vi "Temperature read and control.vi"() -> ()   [LabVIEW 2019]
uses:
  <vilib>/Utility/file.llb/Write Delimited Spreadsheet (DBL).vi
panel:
  in  "Range 2":string(combo)="HI"
  in  "Range1":string(combo)="HI"
  in  "?":enum32{"选项卡 1", "选项卡 2"}(tab)
  out "XY图":cluster{"X":dbl[], "Y":dbl[]}[](graph)
  out "XY图 2":cluster{"X":dbl[], "Y":dbl[]}[](graph)
  in  "EXIT":bool
  in  "LOOP2":dbl=273.15
  out "CHD":dbl
  out "CHC":dbl
  out "CHB":dbl
  in  "控温":bool
  in  "LOOP1":dbl=273.15
  in  "仪器地址":refnum<visa-resource-name>="tcpip0::192.168.1.5::5000::SOCKET"
  out "CHA":dbl
  in  "Delay Time (s)":i32=2 caption="延迟时间(s)"
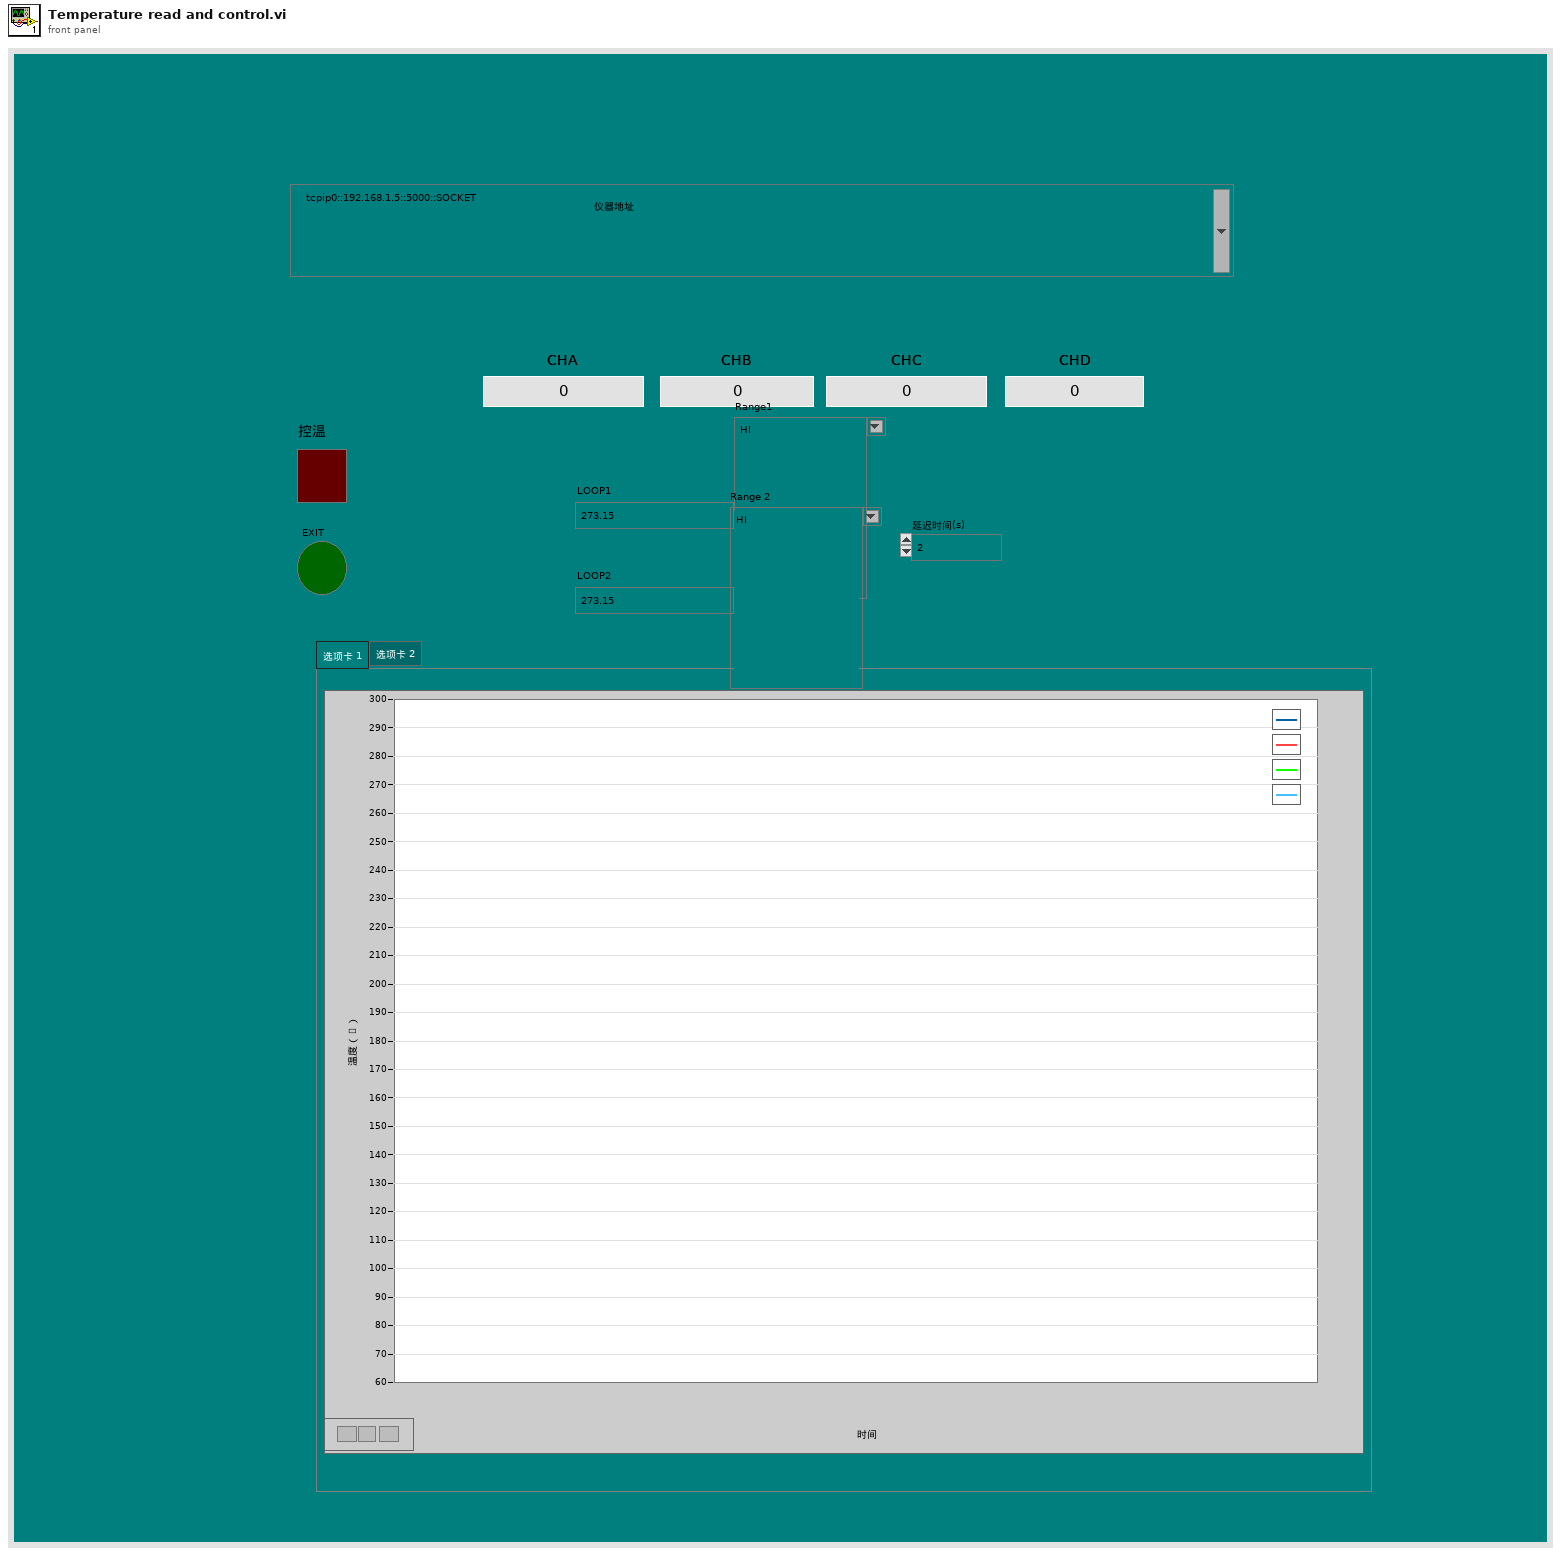
[diagram p1: front panel]
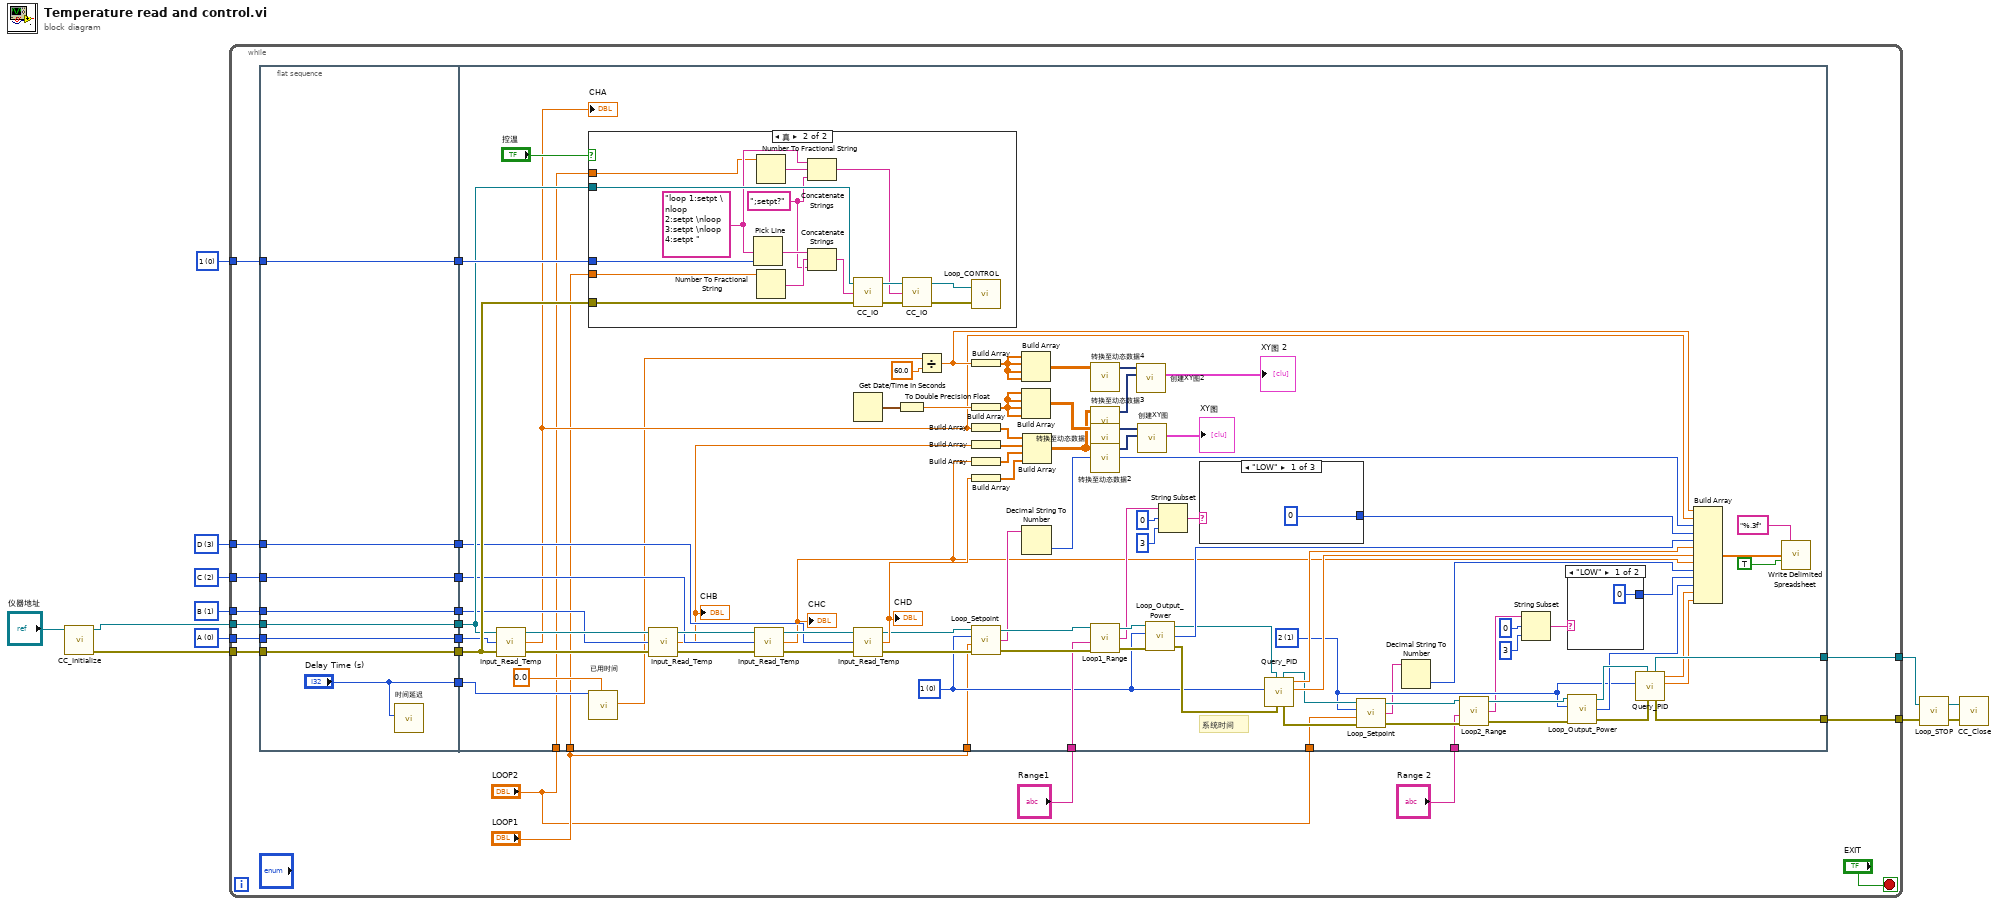
[diagram p0: block diagram]
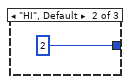
[diagram p2: hidden frame]
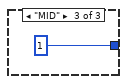
[diagram p3: hidden frame]
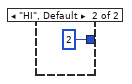
[diagram p4: hidden frame]
diagram:
  w4 = u8 3 items=["A", "B", "C", "D"] ("Input")
  w5 = u8 2 items=["A", "B", "C", "D"] ("Input")
  w6 = u8 1 items=["A", "B", "C", "D"] ("Input")
  w7 = u8 0 items=["A", "B", "C", "D"] ("Input")
  w8 = u8 0 items=["1", "2", "3", "4"] ("Loop")
  n1 = call "CC_Initialize.vi"("VISA resource name"="仪器地址") -> ("error out"=w2:errorcluster, "VISA resource name out"=w3:refnum<visa-resource-name>)  [unwired: 9 in]
  n2 = while {
    tunnel: [w29] -> w11
    tunnel: [w28] -> w12
    tunnel: w3 -> [w30]
    tunnel: w2 -> [w33]
    tunnel: w8 -> [w32]
    tunnel: w7 -> [w31]
    tunnel: w6 -> [w27]
    tunnel: w5 -> [w26]
    tunnel: w4 -> [w25]
    stop <- "EXIT" stop-if-true
    n3 = flat-sequence {
      tunnel: w25 -> [w36]
      tunnel: w26 -> [w37]
      tunnel: w27 -> [w38]
      tunnel: w30 -> [w39]
      tunnel: w31 -> [w40]
      tunnel: w32 -> [w41]
      tunnel: w33 -> [w42]
      tunnel: [w42] -> w24
      tunnel: [w41] -> w23
      tunnel: [w40] -> w22
      tunnel: [w39] -> w21
      tunnel: [w38] -> w20
      tunnel: [w37] -> w19
      tunnel: [w36] -> w18
      tunnel: ["Delay Time (s)"] -> w17
      tunnel: [w76] -> w29
      tunnel: [w75] -> w28
      tunnel: w24 -> [w129]
      tunnel: w23 -> [w128]
      tunnel: w22 -> [w127]
      tunnel: w21 -> [w126]
      tunnel: w20 -> [w119]
      tunnel: w19 -> [w118]
      tunnel: w18 -> [w117]
      tunnel: w17 -> [w99]
      tunnel: "Range1" -> [w86]
      tunnel: "Range 2" -> [w70]
      tunnel: "LOOP2" -> [w48]
      tunnel: "LOOP1" -> [w47]
      tunnel: "LOOP1" -> [w46]
      tunnel: "LOOP2" -> [w45]
      frame #0 {
        n4 = call "时间延迟"("Delay Time (s)"="Delay Time (s)") -> ()  [unwired: 10 in, 1 out]
      }
      frame #1 {
        w65 = u8 1 items=["1", "2", "3", "4"] ("Loop")
        w66 = u8 0 items=["1", "2", "3", "4"] ("Loop")
        # "系统时间"
        n5 = call "Input_Read_Temp.vi"("error in (no error)"=w129, "Input"=w127, "VISA In"=w126) -> ("error out"=w124:errorcluster, "Temperature"=w93:dbl, "VISA Out"=w125:refnum<visa-resource-name>)
        "CHA" <- w93
        n6 = case shown="真" "控温" {
          tunnel: w126 -> [_ w147]
          tunnel: w129 -> [_ w148]
          tunnel: w128 -> [_ w149]
          tunnel: w48 -> [_ w138]
          tunnel: w47 -> [_ w137]
          frame False {
          }
          frame True {
            w145 = ";setpt?" ("string")
            w144 = "loop 1:setpt \nloop 2:setpt \nloop 3:setpt \nloop 4:setpt " ("string")
            n7 = Pick Line(multi-line string=w144, line index=w149) -> (output string=w150:string)  [unwired: 1 in]
            n8 = Number To Fractional String(number=w138) -> (F-format string=w146:string)  [unwired: 3 out]
            n9 = Number To Fractional String(number=w137) -> (F-format string=w151:string)  [unwired: 3 out]
            n10 = Concatenate Strings(w144, w146, w145) -> (w139:string)
            n11 = Concatenate Strings(w150, w151, w145) -> (w152:string)
            n12 = call "CC_IO.vi"("error in (no error)"=w148, "Output Command"=w152, "VISA In"=w147) -> ("error out"=w143:errorcluster, "VISA out"=w142:refnum<visa-resource-name>)  [unwired: 1 out]
            n13 = call "CC_IO.vi"("error in (no error)"=w143, "Output Command"=w139, "VISA In"=w142) -> ("error out"=w140:errorcluster, "VISA out"=w141:refnum<visa-resource-name>)  [unwired: 1 out]
            n14 = call "Loop_CONTROL.vi"("error in (no error)"=w140, "VISA In"=w141) -> ()  [unwired: 2 out]
          }
        }
        n15 = call "已用时间"("Time Target (s)"=w99, "Set Start Time (s)"=0.0) -> ("Elapsed Time (s)"=w63:dbl)  [unwired: 10 in, 7 out]
        n16 = call "Input_Read_Temp.vi"("error in (no error)"=w124, "Input"=w119, "VISA In"=w125) -> ("error out"=w122:errorcluster, "Temperature"=w43:dbl, "VISA Out"=w123:refnum<visa-resource-name>)
        "CHB" <- w43
        n17 = call "Input_Read_Temp.vi"("error in (no error)"=w122, "Input"=w118, "VISA In"=w123) -> ("error out"=w120:errorcluster, "Temperature"=w44:dbl, "VISA Out"=w121:refnum<visa-resource-name>)
        "CHC" <- w44
        n18 = Get Date/Time In Seconds() -> (seconds since 1Jan1904=w131:timestamp)
        n19 = call "Input_Read_Temp.vi"("error in (no error)"=w120, "Input"=w117, "VISA In"=w121) -> ("error out"=w92:errorcluster, "Temperature"=w114:dbl, "VISA Out"=w91:refnum<visa-resource-name>)
        "CHD" <- w114
        n20 = To Double Precision Float(number=w131) -> (double precision float=w109:dbl)
        n21 = Divide(x=w63, y=60.0) -> (x/y=w94:dbl)
        n22 = Build Array(w94) -> (w102:dbl[])
        n23 = Build Array(w109) -> (w108:dbl[])
        n24 = Build Array(w93) -> (w113:dbl[])
        n25 = Build Array(w43) -> (w112:dbl[])
        n26 = Build Array(w44) -> (w111:dbl[])
        n27 = Build Array(w114) -> (w110:dbl[])
        n28 = call "Loop_Setpoint.vi"("VISA in"=w91, "Loop"=w66, "Setpoint"=w46, "error in"=w92) -> ("VISA out"=w90:refnum<visa-resource-name>, "Return"=w62:string, "ErrorOut"=w89:errorcluster)  [unwired: 1 in]
        n29 = Build Array(w102, w102, w102, w102) -> (w103:dbl[][])
        n30 = Build Array(w108, w108, w108, w108) -> (w107:dbl[][])
        n31 = Decimal String To Number(string=w62) -> (number=w61:i32)  [unwired: 2 in, 1 out]
        n32 = Build Array(w113, w112, w111, w110) -> (w104:dbl[][])
        n33 = call "转换至动态数据4"("2D Array"=w103) -> ("Dynamic Data Type"=w105:dynamicdata)  [unwired: 3 in]
        n34 = call "转换至动态数据3"("2D Array"=w104) -> ("Dynamic Data Type"=w106:dynamicdata)  [unwired: 3 in]
        n35 = call "转换至动态数据"("2D Array"=w107) -> ("Dynamic Data Type"=w116:dynamicdata)  [unwired: 3 in]
        n36 = call "转换至动态数据2"("2D Array"=w104) -> ("Dynamic Data Type"=w115:dynamicdata)  [unwired: 3 in]
        n37 = call "Loop1_Range.vi"("VISA in"=w90, "Range"=w86, "error in"=w89) -> ("VISA out"=w88:refnum<visa-resource-name>, "Return"=w54:string, "ErrorOut"=w87:errorcluster)  [unwired: 2 in]
        n38 = call "创建XY图2"("Y Input"=w106, "X Input"=w105) -> ("XY Graph"=→"XY图 2":cluster{"X":dbl[], "Y":dbl[]}[])  [unwired: 8 in, 1 out]
        n39 = call "创建XY图"("Y Input"=w115, "X Input"=w116) -> ("XY Graph"=→"XY图":cluster{"X":dbl[], "Y":dbl[]}[])  [unwired: 8 in, 1 out]
        n40 = call "Loop_Output_Power.vi"("VISA in"=w88, "Loop"=w66, "error in"=w87) -> ("VISA out"=w84:refnum<visa-resource-name>, "Output Pwr (%)"=w85:i32, "ErrorOut"=w83:errorcluster)  [unwired: 2 in]
        n41 = String Subset(string=w54, offset (0)=0 ("偏移量(0)"), length (rest)=3 ("长度（剩余）")) -> (substring=w53:string)
        n42 = case shown="\"LOW\"" w53 {
          tunnel: [0 2 1] -> w57
          frame "LOW" {
          }
          frame "HI", Default {
          }
          frame "MID" {
          }
        }
        n43 = call "Query_PID.vi"("error in (no error)"=w83, "VISA In"=w84, "Output"=w66) -> ("I"=w81:sgl, "P"=w82:sgl, "error out"=w77:errorcluster, "VISA Out"=w78:refnum<visa-resource-name>)  [unwired: 3 in, 2 out]
        n44 = call "Loop_Setpoint.vi"("VISA in"=w78, "Loop"=w65, "Setpoint"=w45, "error in"=w77) -> ("VISA out"=w74:refnum<visa-resource-name>, "Return"=w60:string, "ErrorOut"=w73:errorcluster)  [unwired: 1 in]
        n45 = Decimal String To Number(string=w60) -> (number=w59:i32)  [unwired: 2 in, 1 out]
        n46 = call "Loop2_Range.vi"("VISA in"=w74, "Range"=w70, "error in"=w73) -> ("VISA out"=w72:refnum<visa-resource-name>, "Return"=w49:string, "ErrorOut"=w71:errorcluster)  [unwired: 2 in]
        n47 = String Subset(string=w49, offset (0)=0 ("偏移量(0)"), length (rest)=3 ("长度（剩余）")) -> (substring=w50:string)
        n48 = case shown="\"LOW\"" w50 {
          tunnel: [0 2] -> w58
          frame "LOW" {
          }
          frame "HI", Default {
          }
        }
        n49 = call "Loop_Output_Power.vi"("VISA in"=w72, "Loop"=w65, "error in"=w71) -> ("VISA out"=w80:refnum<visa-resource-name>, "Output Pwr (%)"=w69:i32, "ErrorOut"=w79:errorcluster)  [unwired: 2 in]
        n50 = call "Query_PID.vi"("error in (no error)"=w79, "VISA In"=w80, "Output"=w65) -> ("I"=w67:sgl, "P"=w68:sgl, "error out"=w75:errorcluster, "VISA Out"=w76:refnum<visa-resource-name>)  [unwired: 3 in, 2 out]
        n51 = Build Array(w94, w93, w61, w57, w85, w82, w81, w44, w59, w58, w69, w68, w67) -> (w96:dbl[])
        n52 = call-poly <vilib>:"Write Delimited Spreadsheet.vi"("format (%.3f)"="%.3f", "1D data"=w96, "append to file? (new file:F)"=TRUE) -> ()  [unwired: 11 in, 2 out]
      }
    }
  }
  n53 = call "Loop_STOP.vi"("error in (no error)"=w12, "VISA In"=w11) -> ("error out"=w10:errorcluster, "VISA Out"=w9:refnum<visa-resource-name>)
  n54 = call "CC_Close.vi"("error in (no error)"=w10, "VISA In"=w9) -> ()  [unwired: 1 in, 1 out]
